vi "R_W Serial Data.vi"(8 "error in (no error)":errorcluster, 10 "String In":string, 11 "TE Cooler in":refnum<class "TE Cooler.lvclass">) -> (0 "error out":errorcluster, 2 "String Out":string, 3 "TE Cooler out":refnum<class "TE Cooler.lvclass">)   [LabVIEW 2015, in "TE Cooler.lvlib" / "TE Cooler.lvclass"]
uses:
  TE Cooler.lvclass
  <vilib>/MSR Consulting, LLC/General Reuse/Session APIs/Serial/Serial Session.lvclass
  <vilib>/MSR Consulting, LLC/Devices/Configurable Device/Read Log Session.vi
  <vilib>/MSR Consulting, LLC/General Reuse/Session APIs/Serial/Public/Asynchronous Write.vi
  <vilib>/MSR Consulting, LLC/General Reuse/Session APIs/Serial/Public/Asynchronous Read.vi
  <vilib>/MSR Consulting, LLC/General Reuse/Session APIs/_Session Fwk/Session - Root.lvclass
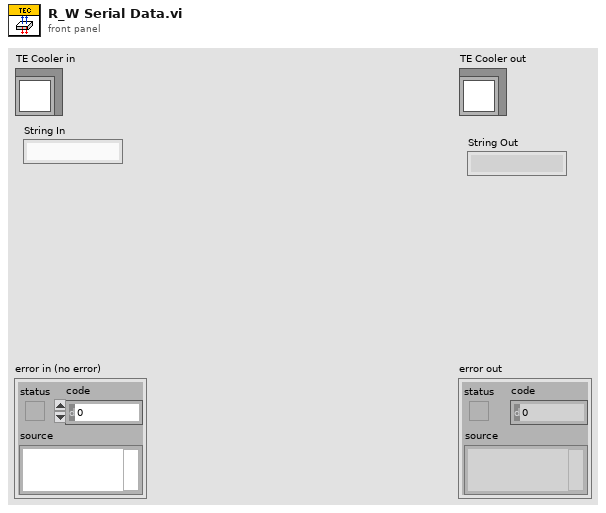
[diagram p1: front panel]
types:
  T1 = typedef "Session - Root.lvclass/Session Handle.ctl" = refnum<data-value>
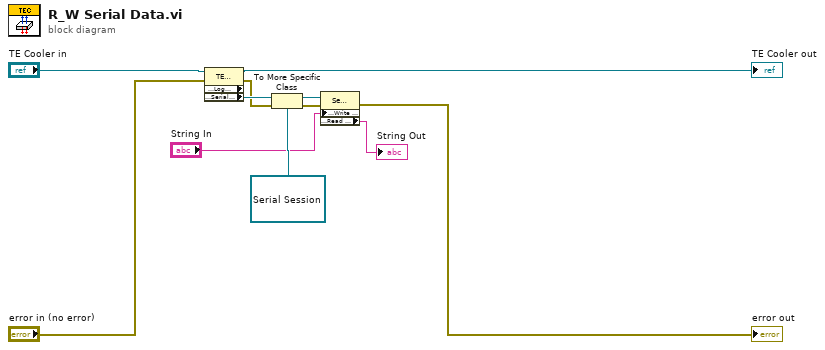
[diagram p0: block diagram]
diagram:
  n1 = property class="TE Tech" props=["Accessors:Log Session", "Accessors:Serial Session"](reference="TE Cooler in", error in="error in (no error)") -> (reference out=→"TE Cooler out":refnum<class "TE Cooler.lvclass">, error out=w7:errorcluster, "Accessors:Serial Session"=w8:T1)  [unwired: 1 out]
  n2 = To More Specific Class(target class=refnum<data-value> refnum, reference=w8, error in=w7) -> (specific class reference=w10:refnum<data-value>, error out=w9:errorcluster)
  n3 = property class="Serial Session"(reference=w10, error in=w9, "Public:Write - Asynchronous"="String In") -> (error out=→"error out":errorcluster, "Public:Read - Asynchronous"=→"String Out":string)  [unwired: 1 out]
